vi "FindChildActorAttributes.vi"(10 "Alias":string, 11 "Actor":refnum<class "Actor.lvclass">) -> (2 "ChildActorAttributes":T1, 3 "Found":bool)   [LabVIEW 2020, in "jettl.lvlib"]
uses:
  jettl.lvlib
  Actor/Actor.lvclass
  Msg/Msg.lvclass
  MsgSet.ctl
  Msg.ctl
  Unified.ctl
  PostSetup.ctl
  PreSetup.ctl
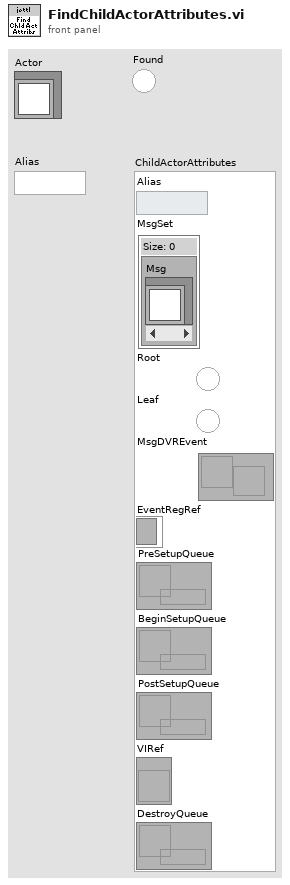
[diagram p1: front panel]
types:
  T1 = typedef "jettl.lvlib/Unified.ctl" = cluster{"Alias":string, "MsgSet":T2, "Root":bool, "Leaf":bool, "MsgDVREvent":refnum<user-event>, "EventRegRef":refnum<event-registration>, "PreSetupQueue":refnum<queue>, "BeginSetupQueue":refnum<queue>, "PostSetupQueue":refnum<queue>, "VIRef":refnum<vi>, "DestroyQueue":refnum<queue>}
  T2 = typedef "jettl.lvlib/MsgSet.ctl" = set{refnum<class "Msg.lvclass">}
  T3 = typedef "jettl.lvlib/ChildUnifiedMap.ctl" = map{string, T1}
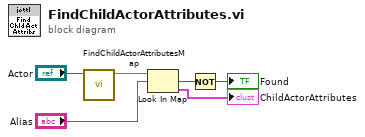
[diagram p0: block diagram]
diagram:
  n1 = call "FindChildActorAttributesMap.vi"("Actor"="Actor") -> ("ChildActorAttributesMap"=w1:T3)  [unwired: 10 in]
  n2 = Look In Map(map=w1, key="Alias") -> (key not found?=w4:bool, value=→"ChildActorAttributes":T1)  [unwired: 1 in]
  n3 = Not(x=w4) -> (.not. x?=→"Found":bool)
